vi "Board Is Space Empty.vi"(8 "error in (no error)":errorcluster, 10 "Coordinate":T1, 11 "Board in":refnum<class "Board.lvclass">) -> (0 "error out":errorcluster, 2 "Empty?":bool, 3 "Board out":refnum<class "Board.lvclass">)   [LabVIEW 2019, in "Board.lvclass"]
uses:
  Board.lvclass
  Food/Food.lvclass
  Player/Player.lvclass
  Snake/Snake.lvclass
  Coordinate STYP.ctl
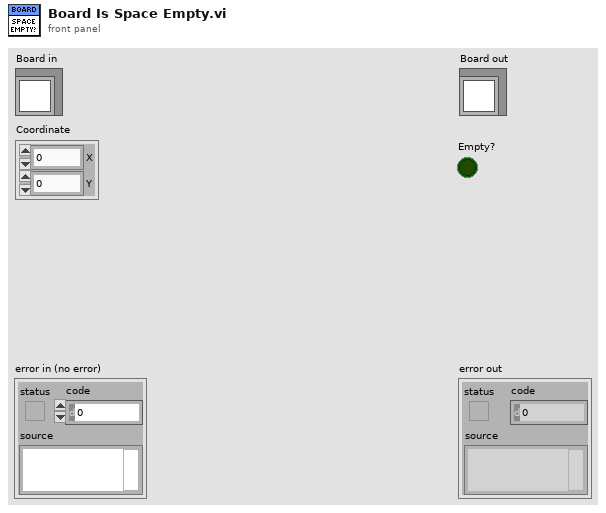
[diagram p1: front panel]
types:
  T1 = typedef "Coordinate STYP.ctl" = cluster{"X":i32, "Y":i32}
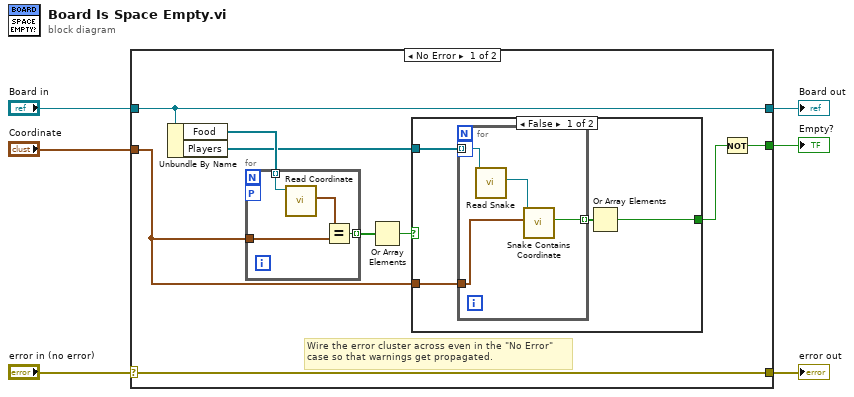
[diagram p0: block diagram]
diagram:
  n1 = case shown="No Error" "error in (no error)" {
    selector: "error in (no error)" -> [w15 w30]
    tunnel: [w15 w30] -> w5
    tunnel: [w14 w29] -> w3
    tunnel: "Board in" -> [w14 w29]
    tunnel: "Coordinate" -> [w9 _]
    tunnel: [w7 _] -> w1
    frame No Error {
      # "Wire the error cluster across even in the \"No Error\"\ncase so that warnings get propagated."
      n2 = Unbundle By Name(w14) -> ("Food"=w13:refnum<class "Food.lvclass">[], "Players"=w11:refnum<class "Player.lvclass">[])
      n3 = for {
        tunnel: w13 -> [w28] mode=indexing
        tunnel: w9 -> [w26]
        tunnel: [w25] -> w12 mode=indexing
        workers-P: _ -> [_]
        n4 = call-dynamic "Read Coordinate.vi"("Food in"=w28) -> ("Coordinate"=w27:T1)  [unwired: 8 in, 2 out]
        n5 = Equal?(x=w27, y=w26) -> (x = y?=w25:bool)
      }
      n6 = Or Array Elements(Boolean array=w12) -> (logical OR=w10:bool)
      n7 = case shown="False" w10 {
        selector: w10 -> [_ w24]
        tunnel: w11 -> [w19 _]
        tunnel: w9 -> [w18 _]
        tunnel: [w16 w24] -> w8
        frame False {
          n8 = for {
            tunnel: w19 -> [w23] mode=indexing
            tunnel: w18 -> [w21]
            tunnel: [w20] -> w17 mode=indexing
            workers-P: _ -> [_]
            n9 = call-dynamic "Read Snake.vi"("Player in"=w23) -> ("Snake.lvclass"=w22:refnum<class "Snake.lvclass">)  [unwired: 8 in, 2 out]
            n10 = call-dynamic "Snake Contains Coordinate.vi"("Coordinate"=w21, "Snake in"=w22) -> ("In Snake?"=w20:bool)  [unwired: 7 in, 2 out]
          }
          n11 = Or Array Elements(Boolean array=w17) -> (logical OR=w16:bool)
        }
        frame True {
        }
      }
      n12 = Not(x=w8) -> (.not. x?=w7:bool)
    }
    frame Error {
    }
  }
  "error out" <- w5
  "Board out" <- w3
  "Empty?" <- w1
